vi "MasterAcquisitionFile_PCO_IOS.vi"() -> ()   [LabVIEW 2020]
uses:
  <userlib>/PCO LabVIEW 5.0.0/pco.camera/Controls/binning.ctl
  <vilib>/vision/driver/IMAQdx.llb/IMAQdx Camera Control Mode.ctl
  <vilib>/vision/driver/IMAQdx.llb/IMAQdx Acquisition Mode.ctl
  <vilib>/userDefined/High Color/IMAQdx.ctl
  <userlib>/PCO LabVIEW 5.0.0/pco.camera/Camera.lvclass
  <vilib>/vision/driver/IMAQdx.llb/IMAQdx Buffer Number Mode.ctl
  <vilib>/DAQmx/write.llb/DAQmx Write (Digital 1D Wfm NChan NSamp).vi
  <vilib>/DAQmx/write.llb/DAQmx Write (Digital Bool 1Line 1Point).vi
  <vilib>/DAQmx/read.llb/DAQmx Read (Analog 1D Wfm NChan NSamp).vi
  <vilib>/Waveform/DWDTOps.llb/DWDT Digital to Boolean Array.vi
  <vilib>/DAQmx/create/channels.llb/DAQmx Create Channel (CO-Pulse Generation-Frequency).vi
  <vilib>/DAQmx/configure/timing.llb/DAQmx Timing (Implicit).vi
  <vilib>/DAQmx/create/channels.llb/DAQmx Create Channel (AI-Voltage-Basic).vi
  <vilib>/DAQmx/configure/timing.llb/DAQmx Timing (Sample Clock).vi
  <vilib>/DAQmx/configure/trigger.llb/DAQmx Start Trigger (Digital Edge).vi
  <vilib>/DAQmx/create/channels.llb/DAQmx Create Channel (DO-Digital Output).vi
  <vilib>/Waveform/DWDTOps.llb/DWDT Boolean Array to Digital.vi
  <vilib>/Waveform/DWDTOps.llb/DWDT Uncompress Digital.vi
  <vilib>/DAQmx/miscellaneous.llb/DAQmx Fill In Error Info.vi
  <vilib>/vision/driver/NI_Vision_Acquisition_Software.lvlib
  <resource>/objmgr/imaqdx.rc
  <resource>/objmgr/daqmx.rc
panel:
  out "Recorded Images":u32=9000
  in  "ROI":cluster{"x0":u64, "y0":u64, "x1":u64, "y1":u64}={"x0"=1, "y0"=1, "x1"=640, "y1"=540}
  in  "Binning":T1={"vert"=4, "horz"=4}
  in  "TriggerMode":T2(ring)=enum."external exposure start"
  in  "Exposure [s]":dbl=0.02 min=0.0005 max=2.0 step=0.001
  out "Image":T3(plugin-control)
  out "LED":bool
  out "Auditory":bool
  out "RPad":bool
  out "LPad":bool
  out "Finished":bool=TRUE
  in  "Generate Stimuli":bool=TRUE
  in  "Sol Stim Parameters":cluster{"Fs":dbl, "Samples":dbl}
  in  "LED Stim Parameters":cluster{"Fs":dbl, "Samples":dbl}
  in  "Sol Duty Cycle (%)":dbl=50.0
  in  "Sol Freq":dbl=1.0
  in  "Sol Dur (s)":dbl=1.0
  in  "LED Duty Cycle (%)":dbl=10.0
  in  "LED Freq":dbl=10.0
  in  "LED Dur (s)":dbl=2.0
  out "Stimulus Order":digitalwaveform[](graph)=[{"t0"=timestamp(0 s since 1904-01-01), "dt"=5e-05, "Y"={"transitions"=[], "data"=array6001000x1[6001000 elements]}}, {"t0"=timestamp(0 s since 1904-01-01), "dt"=5e-05, "Y"={"transitions"=[], "data"=array6001000x1[6001000 elements]}}, {"t0"=timestamp(0 s since 1904-01-01), "dt"=5e-05, "Y"={"transitions"=[], "data"=array6001000x1[6001000 elements]}}, {"t0"=timestamp(0 s since 1904-01-01), "dt"=5e-05, "Y"={"transitions"=[], "data"=array6001000x1[6001000 elements]}}]
  out "Solenoid Stim":digitalwaveform(graph)={"t0"=timestamp(0 s since 1904-01-01), "dt"=5e-05, "Y"={"transitions"=[], "data"=array20000x1[20000 elements]}}
  in  "Trial Offset (s)":dbl=15.0
  in  "Interstim (s)":dbl=30.0
  in  "Right Pad":dbl=1.0
  in  "Left Pad":dbl=1.0
  in  "Auditory":dbl=1.0
  in  "LED":dbl
  out "?":T3(plugin-control)
  out "?":T3(plugin-control)
  out "?":T3(plugin-control)
  in  "stop":bool
  out "PCO":bool=TRUE
  out "Pupil Cam":bool=TRUE
  out "Whisk Cam":bool=TRUE
  out "Web Cam":bool=TRUE
  out "Analog":bool=TRUE
  out "Web Cam Fs":dbl(knob)=16.167664670658684 scale=0.0..200.0
  out "Whisk Cam Fs":dbl(knob)=150.0 scale=0.0..200.0
  out "Last Whisk\nBuffer 2":u32=9001
  out "Pupil Cam Fs":dbl(knob)=30.0 scale=0.0..200.0
  out "Dropped 2":u32(slide) caption="Pupil Cam" scale=0.0..99.0
  out "Dev1 Samples":i32=6000014
  in  "Dev1 Analog Channels":string[](array[string])=["Cortical_LH", "Force_Sensor", "LPadSol", "RPadSol", "AudSol", "Hippocampus", "EMG", "Cortical_RH", "OptoLED"]
  in  "Analog Acquisition":cluster{"Analog Fs":u16}={"Analog Fs"=20000} {"Analog Fs" format="%0.0f"}
  in  "Sampling Rates":T4={"CBV Cam Fs"=30, "Whisk Cam Fs"=150, "Web Cam Fs"=30, "Pupil Cam Fs"=30}
  out "Notes Size":i32=10
  out "Notes Reversed":string[](array[string])=["Experimenter", "Animal ID", "Hemisphere", "Solenoid PSI", "Isoflurane time", "Session ID", "Amplifier Gain", "Opto LED (mW)", "Wavelengths", "Lens mag"]
  out "Notes Array":string[](array[string])=["Lens mag", "Wavelengths", "Opto LED (mW)", "Amplifier Gain", "Session ID", "Isoflurane time", "Solenoid PSI", "Hemisphere", "Animal ID", "Experimenter"]
  in  "Notes:":T5={"Experimenter"="Kevin", "Animal ID"="FS28", "Hemisphere"="RH", "Solenoid PSI"="10", "Isoflurane time"="1320", "Session ID"="Imaging Session Two", "Amplifier Gain"="10000", "Opto LED (mW)"="10", "Wavelengths"="RGB", "Lens mag"="3X"}
  in  "Target Path":path=path "D:/FS28/1min_470_OptoLED_NotesTests" caption="Final Save Location"
  out "Dropped":u32(slide) caption="Whisk Cam" scale=0.0..999.0
  out "Filename":string="230407_13_50_46"
  out "CBV Camera":bool=TRUE
  out "Time Elapsed (Min)":cluster{dbl, dbl}(slide)={5.0, 5.0012167100000005} scale=0.0..15.0 scale format="%.1g"
  in  "Time (min)":dbl(knob)=5.0 min=0.5 max=20.0 step=0.5 scale=0.0..20.0 scale format="%#_2g"
  in  "Temp Path":path=path "D:/LabVIEW Streamed Data" caption="Temporary Path for Streamed Data"
  out "Last Whisk\nBuffer":u32=45001
  # "PCO Parameters"
  # "Stimuli"
  # "LPAD"
  # "RPAD"
  # "AUD"
  # "LED"
  # "Dropped Frames"
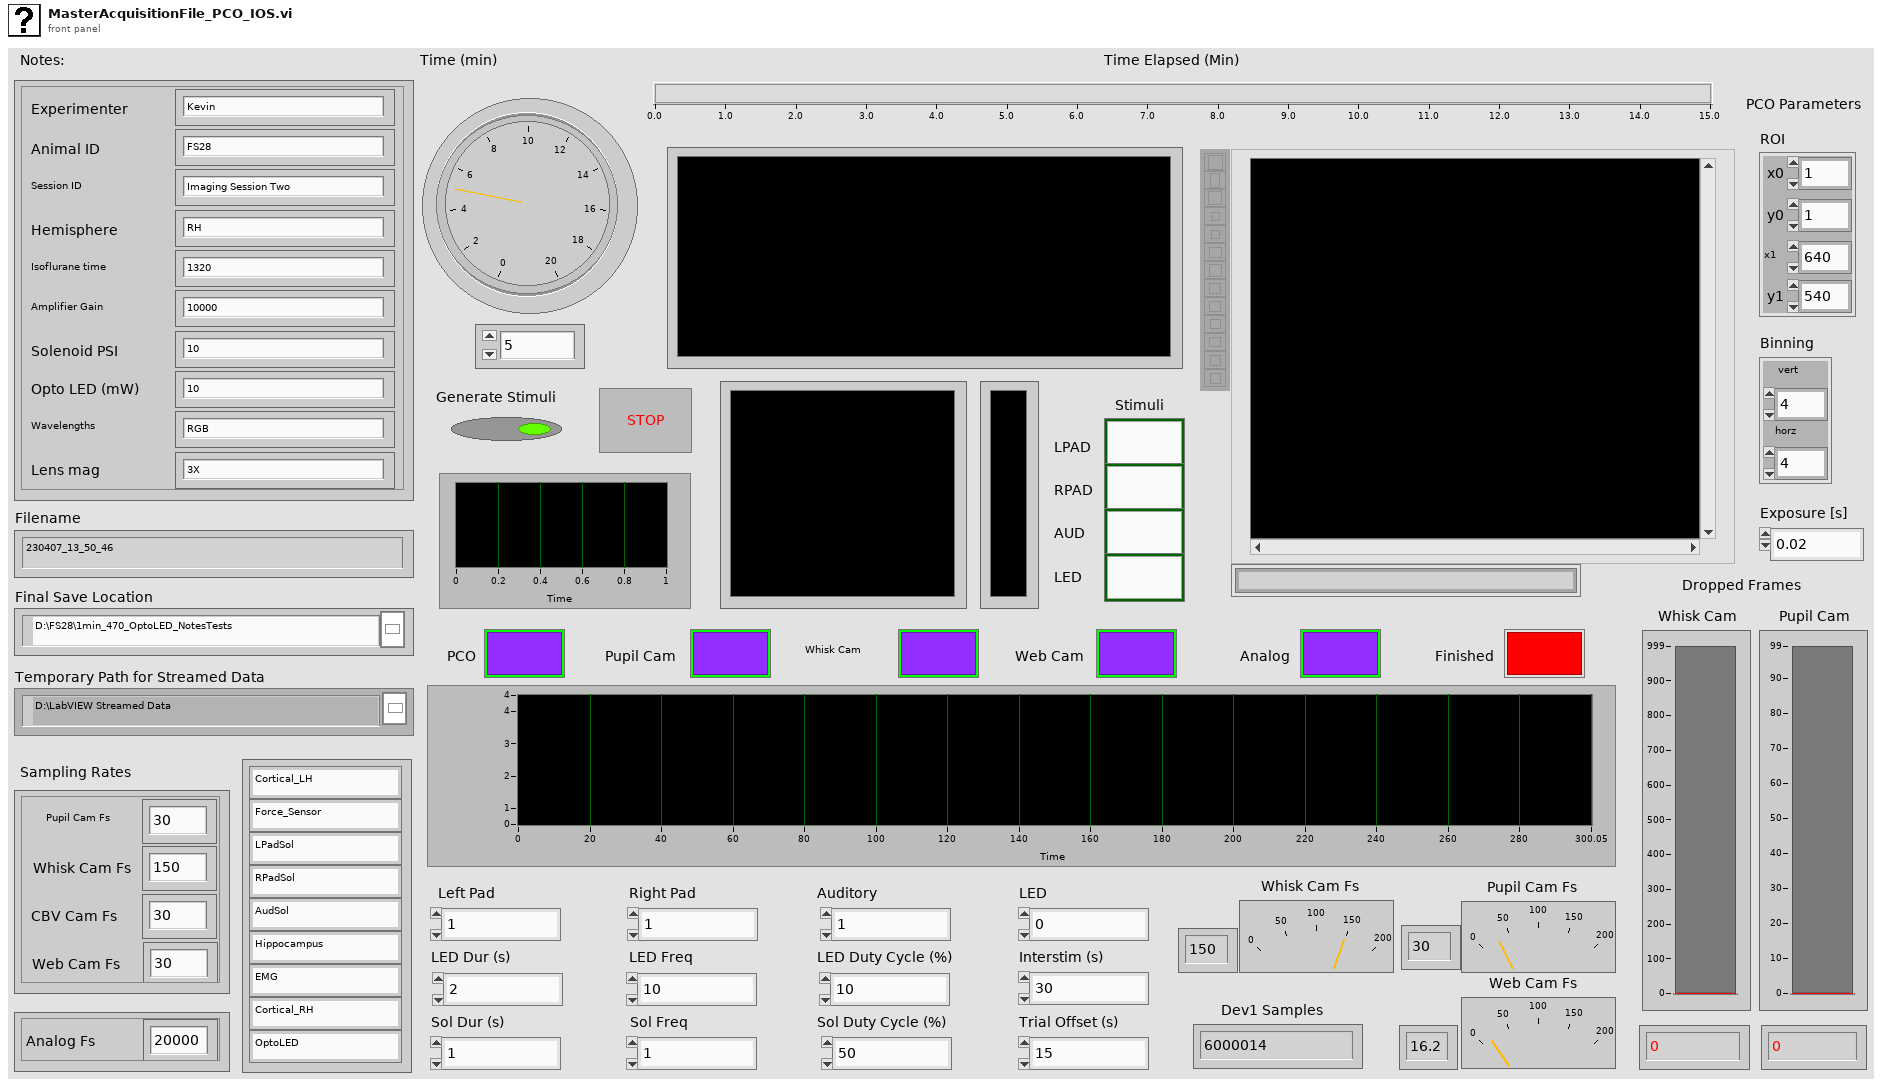
[diagram p1: front panel]
types:
  T1 = typedef "Camera.lvclass/binning.ctl" = cluster{"vert":u16, "horz":u16}
  T2 = enum16{"auto sequence", "software trigger", "external exposure start", "external exposure control"}
  T3 = typedef "IMAQ Image.ctl" = refnum<image>
  T4 = cluster{"CBV Cam Fs":u16, "Whisk Cam Fs":u16, "Web Cam Fs":u16, "Pupil Cam Fs":u16}
  T5 = cluster{"Experimenter":string, "Animal ID":string, "Hemisphere":string, "Solenoid PSI":string, "Isoflurane time":string, "Session ID":string, "Amplifier Gain":string, "Opto LED (mW)":string, "Wavelengths":string, "Lens mag":string}
  T6 = typedef "Image Type" = u32
  T7 = typedef "IMAQdx.ctl" = refnum<k21>
  T8 = enum16{"open", "replace", "create", "open or create", "replace or create", "replace or create with confirmation"}
  T9 = typedef "NI_Vision_Acquisition_Software.lvlib/IMAQdx Acquisition Mode.ctl" = enum32{"One Shot", "Continuous"}
  T10 = typedef "NI_Vision_Acquisition_Software.lvlib/IMAQdx Camera Control Mode.ctl" = enum32{"Controller", "Listener"}
  T11 = enum16{"open", "open or create", "create or replace", "create", "open (read-only)"}
  T12 = cluster{"exposure_time_s":dbl, "delay_time_s":dbl, "roi":cluster{"x0":u64, "y0":u64, "x1":u64, "y1":u64}, "timestamp_mode":u16, "pixelrate":u32, "trigger_mode":u16, "acquire_mode":u16, "metadata_mode":u16, "noisefilter_mode":u16, "binning":T1}
  T13 = typedef "IMAQ AVI2 Refnum.ctl" = refnum<k20>
  T14 = enum16{"sequence", "sequence non blocking", "ring buffer", "fifo", "sequence_dpcore", "sequence_non_blocking_dpcore", "ring_buffer_dpcore", "fifo_dpcore", "tif", "multitif", "pcoraw", "b16", "dicom", "multidicom"}
  T15 = enum16{"Undefined", "Mono8", "Mono16", "BGRA8", "RGBA8", "BGRA16", "RGBA16", "CompressedMono8"}
  T16 = enum16{"big-endian, network order", "native, host order", "little-endian"}
  T17 = typedef "NI_Vision_Acquisition_Software.lvlib/IMAQdx Buffer Number Mode.ctl" = enum32{"Next", "Last", "Buffer Number", "Every", "Last New"}
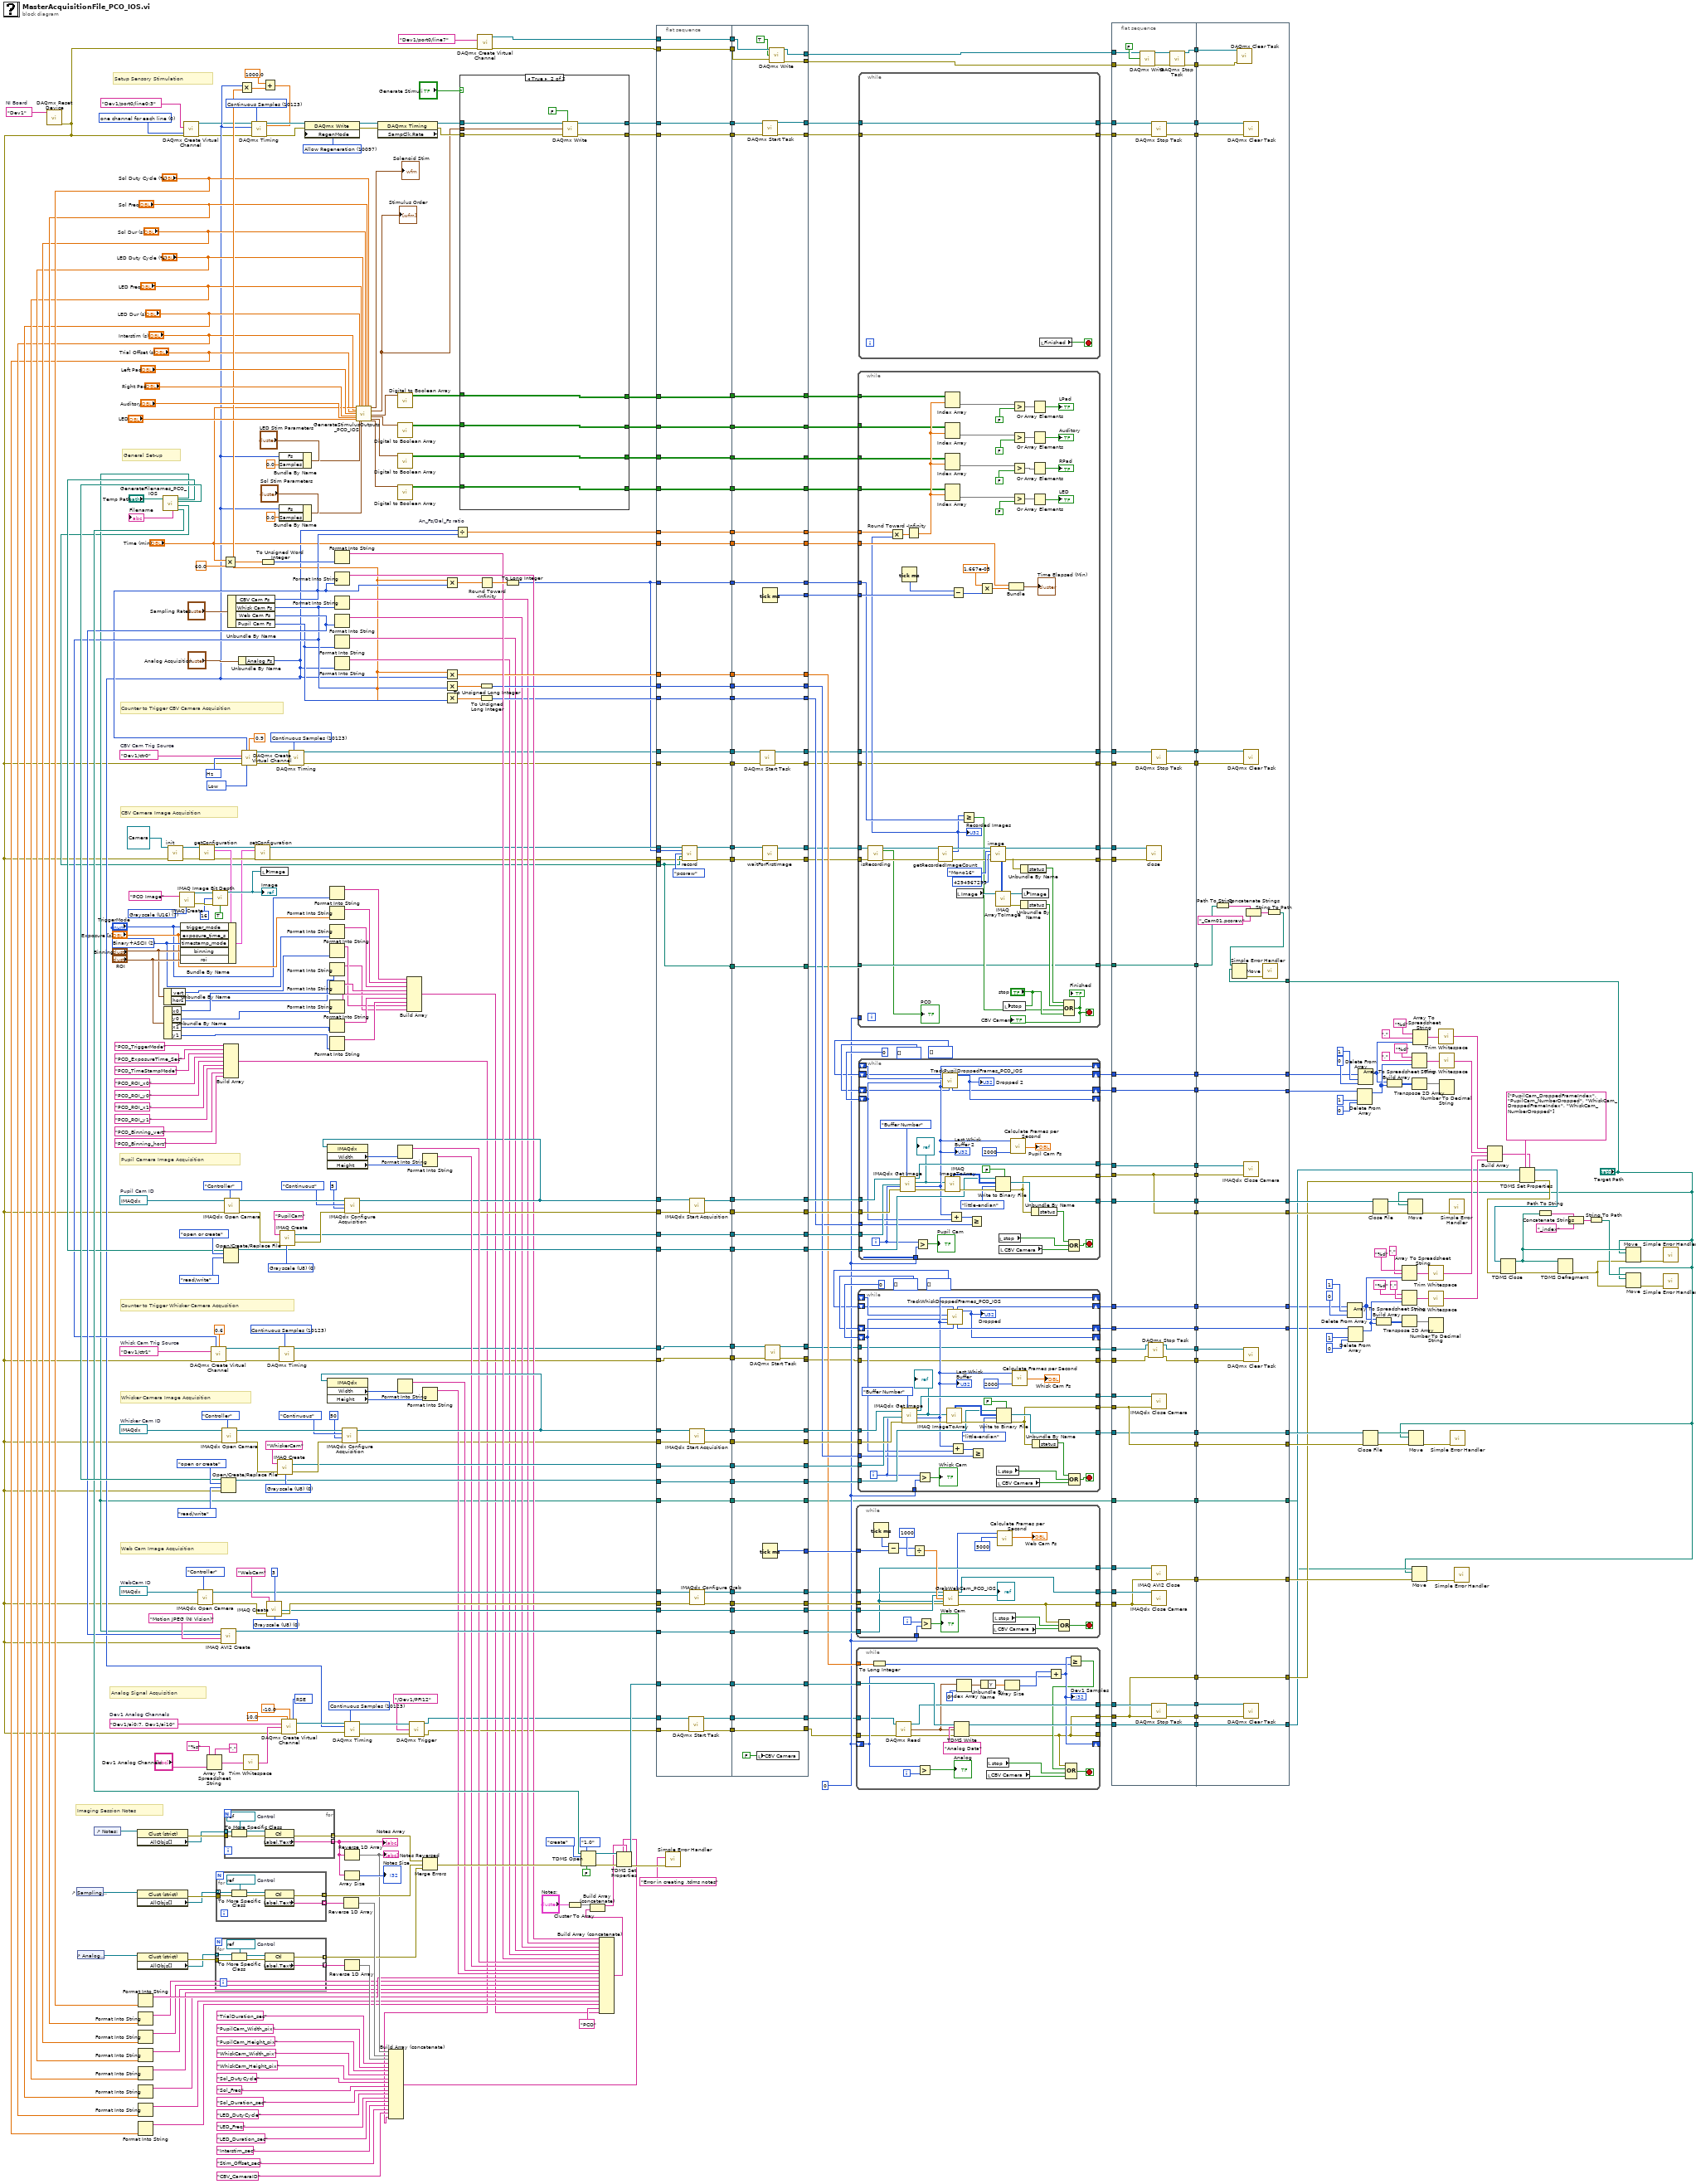
[diagram p0: block diagram]
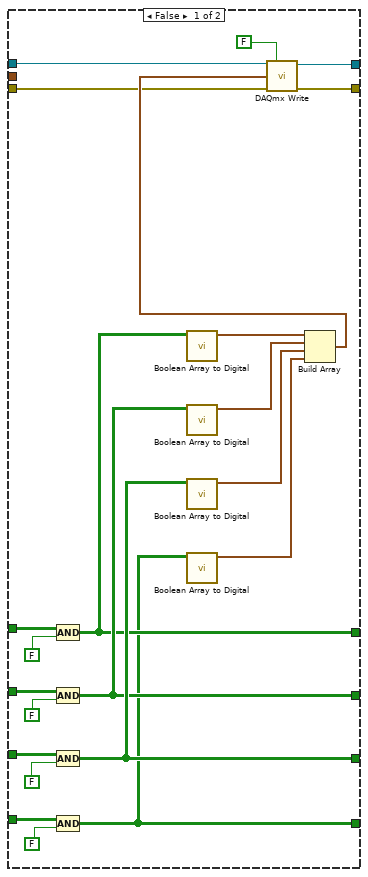
[diagram p2: hidden frame]
diagram:
  w6 = u16 2 items=["OFF", "Binary", "Binary+ASCII", "ASCII"] ("wTimeStampMode")
  w98 = T6 7 items=["Grayscale (U8)", "Grayscale (I16)", "Grayscale (SGL)", "Complex (CSG)", "RGB (U32)", "HSL (U32)", "RGB (U64)", "Grayscale (U16)"] ("Image Type")
  w179 = 10097 items=["Allow Regeneration"=10097, "Do Not Allow Regeneration"=10158] ("RegenMode")
  w180 = 10123 items=["Finite Samples"=10178, "Continuous Samples"=10123, "Hardware Timed Single Point"=12522] ("sample mode")
  w183 = 0 items=["one channel for each line", "one channel for all lines"] ("line grouping")
  w352 = tag "Dev1/ai0:7, Dev1/ai10"  # Dev1 Analog Channels
  w355 = T7 "cam3"  # WebCam ID
  w341 = T7 "cam1"  # Whisker Cam ID
  w461 = tag "Dev1/ctr1"  # Whisk Cam Trig Source
  w303 = T7 "cam2"  # Pupil Cam ID
  w152 = tag "Dev1/ctr0"  # CBV Cam Trig Source
  w306 = T6 0 items=["Grayscale (U8)", "Grayscale (I16)", "Grayscale (SGL)", "Complex (CSG)", "RGB (U32)", "HSL (U32)", "RGB (U64)", "Grayscale (U16)"] ("Image Type")
  w236 = 0
  w410 = 10123 items=["Finite Samples"=10178, "Continuous Samples"=10123, "Hardware Timed Single Point"=12522] ("sample mode")
  w413 = 10083 items=["default"=-1, "RSE"=10083, "NRSE"=10078, "Differential"=10106, "Pseudodifferential"=12529] ("input terminal configuration")
  w444 = T6 0 items=["Grayscale (U8)", "Grayscale (I16)", "Grayscale (SGL)", "Complex (CSG)", "RGB (U32)", "HSL (U32)", "RGB (U64)", "Grayscale (U16)"] ("Image Type")
  w451 = tag "Dev1"  # NI Board
  w452 = 10123 items=["Finite Samples"=10178, "Continuous Samples"=10123, "Hardware Timed Single Point"=12522] ("sample mode")
  w455 = 10373 items=["Hz"=10373] ("units")
  w456 = 10214 items=["High"=10192, "Low"=10214] ("idle state")
  w457 = 10123 items=["Finite Samples"=10178, "Continuous Samples"=10123, "Hardware Timed Single Point"=12522] ("sample mode")
  w464 = T6 0 items=["Grayscale (U8)", "Grayscale (I16)", "Grayscale (SGL)", "Complex (CSG)", "RGB (U32)", "HSL (U32)", "RGB (U64)", "Grayscale (U16)"] ("Image Type")
  # "General Set-up"
  # "Pupil Camera Image Acquisition"
  # "Whisker Camera Image Acquisition"
  # "Imaging Session Notes"
  # "Setup Sensory Stimulation"
  # "CBV Camera Image Acquisition"
  # "Counter to Trigger CBV Camera Acquisition"
  # "Counter to Trigger Whisker Camera Acqusition"
  # "Web Cam Image Acquisition"
  # "Analog Signal Acquisition"
  n1 = call <vilib>:"DAQmx Reset Device.vi"("device in"=w451) -> ("error out"=w60:errorcluster)  [unwired: 14 in]
  n2 = control-ref of="Sampling Rates"() -> (w361:refnum<vi>)
  n3 = control-ref of="Analog Acquisition"() -> (w360:refnum<vi>)
  n4 = control-ref of="Notes:"() -> (w382:refnum<vi>)
  n5 = property class="Clust (strict)"(reference=w382) -> (error out=w385:errorcluster, "AllObjs[]"=w319:refnum<vi>[])  [unwired: 1 in, 1 out]
  n6 = property class="Clust (strict)"(reference=w361) -> (error out=w380:errorcluster, "AllObjs[]"=w320:refnum<vi>[])  [unwired: 1 in, 1 out]
  n7 = property class="Clust (strict)"(reference=w360) -> (error out=w359:errorcluster, "AllObjs[]"=w318:refnum<vi>[])  [unwired: 1 in, 1 out]
  n8 = Format Into String("Sol Duty Cycle (%)") -> (resulting string=w213:string)  [unwired: 3 in, 1 out]
  n9 = Format Into String("Sol Freq") -> (resulting string=w212:string)  [unwired: 3 in, 1 out]
  n10 = Format Into String("Sol Dur (s)") -> (resulting string=w211:string)  [unwired: 3 in, 1 out]
  n11 = Format Into String("LED Duty Cycle (%)") -> (resulting string=w210:string)  [unwired: 3 in, 1 out]
  n12 = Format Into String("LED Freq") -> (resulting string=w209:string)  [unwired: 3 in, 1 out]
  n13 = Format Into String("LED Dur (s)") -> (resulting string=w208:string)  [unwired: 3 in, 1 out]
  n14 = Format Into String("Interstim (s)") -> (resulting string=w207:string)  [unwired: 3 in, 1 out]
  n15 = Format Into String("Trial Offset (s)") -> (resulting string=w206:string)  [unwired: 3 in, 1 out]
  n16 = call "GenerateFilenames_PCO_IOS.vi"("path"="Temp Path") -> ("TDMS Path"=w377:path, "PCO Path"=w68:path, "Basler Path"=w447:path, "WebCam Path"=w102:path, "Analog file name"=→"Filename":string, "Basler2 Path"=w302:path)  [unwired: 3 in, 2 out]
  n17 = Unbundle By Name("Binning") -> ("vert"=w7:u16, "horz"=w8:u16)
  n18 = Unbundle By Name("ROI") -> ("x0"=w9:u64, "y0"=w10:u64, "x1"=w11:u64, "y1"=w12:u64)
  n19 = call-dynamic "init.vi"("Camera in"=refnum<class "Camera.lvclass"> refnum ("PCOCamera in"), "error in (no error)"=w60) -> ("Camera out"=w91:refnum<class "Camera.lvclass">, "error out"=w90:errorcluster)  [unwired: 7 in]
  n20 = call "IMAQ Create"("Image Name"="PCO Image", "Image Type"=w98) -> ("New Image"=w97:T3, "error out"=w96:errorcluster)  [unwired: 3 in]
  n21 = call-poly <vilib>:"DAQmx Create Virtual Channel.vi"("lines"=tag "Dev1/port0/line0:3", "line grouping"=w183, "error in"=w60) -> ("task out"=w182:refnum<k21>, "error out"=w181:errorcluster)  [unwired: 11 in]
  n22 = call <vilib>:"IMAQdx Open Camera.vi"("Camera Control Mode"=IMAQdx_Camera_Control_Mode."Controller", "error in"=w60, "Session In"=w355) -> ("error out"=w440:errorcluster, "Session Out"=w438:T7)  [unwired: 7 in]
  n23 = call-dynamic "getConfiguration.vi"("error in (no error)"=w90, "Camera in"=w91) -> ("error out"=w89:errorcluster, "configuration"=w93:T12, "Camera out"=w92:refnum<class "Camera.lvclass">)  [unwired: 7 in]
  n24 = Bundle By Name(cluster=w93, "trigger_mode"="TriggerMode", "exposure_time_s"="Exposure [s]", "timestamp_mode"=w6, "binning"="Binning", "roi"="ROI") -> (w88:T12)
  n25 = Array To Spreadsheet String(delimiter (Tab)=",", array="Dev1 Analog Channels", 3:"%s" ("format string")) -> (spreadsheet string=w349:string)
  n26 = call "IMAQ Image Bit Depth"("Image"=w97, "Bit Depth (0)"=u32 16, "error in (no error)"=w96, "Get/Set Bit Depth? (Set)"=TRUE) -> ("Image Out"=w99:T3)  [unwired: 9 in, 2 out]
  "Image" <- w99
  n27 = for {
    tunnel: [w476] -> w357 mode=indexing
    tunnel: w359 -> [w475]
    tunnel: [w473] -> w358 mode=indexing
    tunnel: w318 -> [w472] mode=indexing
    w477 = refnum<vi> refnum  # Control
    n28 = To More Specific Class(target class=w477, reference=w472, error in=w475) -> (specific class reference=w478:refnum<vi>, error out=w474:errorcluster)
    n29 = property class="Ctl"(reference=w478, error in=w474) -> (error out=w473:errorcluster, "Label.Text"=w476:string)  [unwired: 1 out]
  }
  n30 = for {
    tunnel: [w483] -> w381 mode=indexing
    tunnel: w380 -> [w482]
    tunnel: [w480] -> w367 mode=indexing
    tunnel: w320 -> [w479] mode=indexing
    w484 = refnum<vi> refnum  # Control
    n31 = To More Specific Class(target class=w484, reference=w479, error in=w482) -> (specific class reference=w485:refnum<vi>, error out=w481:errorcluster)
    n32 = property class="Ctl"(reference=w485, error in=w481) -> (error out=w480:errorcluster, "Label.Text"=w483:string)  [unwired: 1 out]
  }
  n33 = Open/Create/Replace File(file path (use dialog)=w447, error in=w60, operation (0:open)=T8."open or create", access (0:read/write)=enum16{"read/write", "read-only", "write-only"}."read/write") -> (refnum out=w419:refnum<file>)  [unwired: 2 in, 2 out]
  n34 = call <vilib>:"IMAQdx Open Camera.vi"("Camera Control Mode"=IMAQdx_Camera_Control_Mode."Controller", "error in"=w60, "Session In"=w341) -> ("error out"=w467:errorcluster, "Session Out"=w470:T7)  [unwired: 7 in]
  n35 = Multiply(x="Time (min)", y=60.0) -> (x*y=w223:dbl)
  n36 = Build Array("PCO_TriggerMode", "PCO_ExposureTime_Sec", "PCO_TimeStampMode", "PCO_ROI_x0", "PCO_ROI_y0", "PCO_ROI_x1", "PCO_ROI_y1", "PCO_Binning_vert", "PCO_Binning_horz") -> (w20:string[])
  n37 = Open/Create/Replace File(file path (use dialog)=w302, operation (0:open)=T8."open or create", access (0:read/write)=enum16{"read/write", "read-only", "write-only"}."read/write") -> (refnum out=w287:refnum<file>)  [unwired: 3 in, 2 out]
  n38 = call <vilib>:"IMAQdx Open Camera.vi"("Camera Control Mode"=IMAQdx_Camera_Control_Mode."Controller", "error in"=w60, "Session In"=w303) -> ("error out"=w309:errorcluster, "Session Out"=w312:T7)  [unwired: 7 in]
  n39 = for {
    tunnel: [w490] -> w384 mode=indexing
    tunnel: w385 -> [w489]
    tunnel: [w487] -> w368 mode=indexing
    tunnel: w319 -> [w486] mode=indexing
    w491 = refnum<vi> refnum  # Control
    n40 = To More Specific Class(target class=w491, reference=w486, error in=w489) -> (specific class reference=w492:refnum<vi>, error out=w488:errorcluster)
    n41 = property class="Ctl"(reference=w492, error in=w488) -> (error out=w487:errorcluster, "Label.Text"=w490:string)  [unwired: 1 out]
  }
  "Notes Array" <- w384
  n42 = Unbundle By Name("Sampling Rates") -> ("CBV Cam Fs"=w224:u16, "Whisk Cam Fs"=w276:u16, "Web Cam Fs"=w354:u16, "Pupil Cam Fs"=w270:u16)
  n43 = call-poly <vilib>:"DAQmx Create Virtual Channel.vi"("frequency"=w276, "duty cycle"=0.6, "counter"=w461, "error in"=w60) -> ("task out"=w459:refnum<k21>, "error out"=w458:errorcluster)  [unwired: 10 in]
  n44 = call "IMAQ AVI2 Create"("error in (no error)"=w60, "Codec"="Motion JPEG (NI Vision)", "Frames Per Second"=w354, "AVI Path"=w102) -> ("AVI Refnum"=w430:T13)  [unwired: 6 in, 1 out]
  n45 = Unbundle By Name("Analog Acquisition") -> ("Analog Fs"=w196:u16)
  n46 = Multiply(x=w196, y=w223) -> (x*y=w161:dbl)
  n47 = call-poly <vilib>:"DAQmx Create Virtual Channel.vi"("frequency"=w224, "duty cycle"=0.9, "counter"=w152, "units"=w455, "error in"=w60, "idle state"=w456) -> ("task out"=w454:refnum<k21>, "error out"=w453:errorcluster)  [unwired: 8 in]
  n48 = call <vilib>:"Trim Whitespace.vi"("string"=w349) -> ("trimmed string"=w348:string)  [unwired: 1 in]
  n49 = call-dynamic "setConfiguration.vi"("error in (no error)"=w89, "configuration"=w88, "Camera in"=w92) -> ("error out"=w72:errorcluster, "Camera out"=w71:refnum<class "Camera.lvclass">)  [unwired: 7 in]
  n50 = To Unsigned Word Integer(number=w223) -> (unsigned 16bit integer=w344:u16)
  n51 = local write "Image"(w99) -> ()
  n52 = Add(x=1000.0, y=w161) -> (x+y=w159:dbl)
  n53 = call-poly <vilib>:"DAQmx Timing.vi"("task/channels in"=w182, "sample mode"=w180, "samples per channel"=w159, "rate"=w196, "error in"=w181) -> ("task out"=w176:refnum<k21>, "error out"=w175:errorcluster)  [unwired: 9 in]
  n54 = call "IMAQ Create"("Border Size"=3, "Image Name"="WebCam", "Image Type"=w444, "error in (no error)"=w440) -> ("New Image"=w437:T3, "error out"=w439:errorcluster)  [unwired: 1 in]
  n55 = call "IMAQ Create"("Image Name"="WhiskerCam", "Image Type"=w464, "error in (no error)"=w467) -> ("New Image"=w339:T3, "error out"=w465:errorcluster)  [unwired: 2 in]
  n56 = Bundle By Name(cluster="LED Stim Parameters", "Fs"=w196, "Samples"=0.0) -> (w229:cluster{"Fs":dbl, "Samples":dbl})
  n57 = Bundle By Name(cluster="Sol Stim Parameters", "Fs"=w196, "Samples"=0.0) -> (w230:cluster{"Fs":dbl, "Samples":dbl})
  n58 = call-poly <vilib>:"DAQmx Timing.vi"("task/channels in"=w459, "sample mode"=w457, "error in"=w458) -> ("task out"=w35:refnum<k21>, "error out"=w37:errorcluster)  [unwired: 11 in]
  n59 = call "IMAQ Create"("Image Name"="PupilCam", "Image Type"=w306, "error in (no error)"=w309) -> ("New Image"=w279:T3, "error out"=w307:errorcluster)  [unwired: 2 in]
  n60 = call-poly <vilib>:"DAQmx Create Virtual Channel.vi"("maximum value"=10.0, "minimum value"=-10.0, "input terminal configuration"=w413, "physical channels"=w352, "name to assign"=w348, "error in"=w60) -> ("task out"=w412:refnum<k21>, "error out"=w411:errorcluster)  [unwired: 8 in]
  n61 = call-poly <vilib>:"DAQmx Timing.vi"("task/channels in"=w454, "sample mode"=w452, "error in"=w453) -> ("task out"=w44:refnum<k21>, "error out"=w42:errorcluster)  [unwired: 11 in]
  n62 = property class="DAQmx Write"(reference=w176, error in=w175, "RegenMode"=w179) -> (reference out=w177:refnum<k21>, error out=w178:errorcluster)
  n63 = Format Into String("TriggerMode") -> (resulting string=w19:string)  [unwired: 3 in, 1 out]
  n64 = Format Into String("Exposure [s]") -> (resulting string=w18:string)  [unwired: 3 in, 1 out]
  n65 = Format Into String(w6) -> (resulting string=w17:string)  [unwired: 3 in, 1 out]
  n66 = Format Into String(w7) -> (resulting string=w2:string)  [unwired: 3 in, 1 out]
  n67 = Format Into String(w8) -> (resulting string=w1:string)  [unwired: 3 in, 1 out]
  n68 = Format Into String(w9) -> (resulting string=w16:string)  [unwired: 3 in, 1 out]
  n69 = Format Into String(w10) -> (resulting string=w15:string)  [unwired: 3 in, 1 out]
  n70 = Format Into String(w11) -> (resulting string=w14:string)  [unwired: 3 in, 1 out]
  n71 = Format Into String(w12) -> (resulting string=w13:string)  [unwired: 3 in, 1 out]
  n72 = Format Into String(w344) -> (resulting string=w346:string)  [unwired: 3 in, 1 out]
  n73 = Format Into String(w224) -> (resulting string=w274:string)  [unwired: 3 in, 1 out]
  n74 = Format Into String(w276) -> (resulting string=w273:string)  [unwired: 3 in, 1 out]
  n75 = Format Into String(w354) -> (resulting string=w272:string)  [unwired: 3 in, 1 out]
  n76 = Format Into String(w270) -> (resulting string=w241:string)  [unwired: 3 in, 1 out]
  n77 = Format Into String(w196) -> (resulting string=w240:string)  [unwired: 3 in, 1 out]
  n78 = call <vilib>:"IMAQdx Configure Acquisition.vi"("error in"=w465, "Number of Buffers"=u32 50, "Continuous?"=IMAQdx_Acquisition_Mode."Continuous", "Session In"=w470) -> ("error out"=w248:errorcluster, "Session Out"=w340:T7)  [unwired: 6 in]
  n79 = property class="IMAQdx"(reference=w340) -> ("Width"=w343:u32, "Height"=w342:u32)  [unwired: 1 in, 2 out]
  n80 = Reverse 1D Array(array=w381) -> (reversed array=w371:string[])
  n81 = Reverse 1D Array(array=w384) -> (reversed array=w317:string[])
  "Notes Reversed" <- w317
  n82 = Array Size(array=w384) -> (size(s)=→"Notes Size":i32)
  n83 = Reverse 1D Array(array=w357) -> (reversed array=w356:string[])
  n84 = call <vilib>:"IMAQdx Configure Acquisition.vi"("error in"=w307, "Number of Buffers"=u32 5, "Continuous?"=IMAQdx_Acquisition_Mode."Continuous", "Session In"=w312) -> ("error out"=w289:errorcluster, "Session Out"=w280:T7)  [unwired: 6 in]
  n85 = property class="IMAQdx"(reference=w280) -> ("Width"=w301:u32, "Height"=w300:u32)  [unwired: 1 in, 2 out]
  n86 = call-poly <vilib>:"DAQmx Timing.vi"("task/channels in"=w412, "sample mode"=w410, "rate"=w196, "error in"=w411) -> ("task out"=w316:refnum<k21>, "error out"=w409:errorcluster)  [unwired: 10 in]
  n87 = call "GenerateStimulusOutputs_PCO_IOS.vi"("Trial duration (min)"="Time (min)", "Rest duration(s)"="Interstim (s)", "trial offset (s)"="Trial Offset (s)", "Left Pad"="Left Pad", "Right Pad"="Right Pad", "Auditory"="Auditory", "LED"="LED", "LED Stim Duration (s)"="LED Dur (s)", "LED Stim Parameters"=w229, "LED Frequency"="LED Freq", "Sol Stim Parameters"=w230, "LED duty cycle (%)"="LED Duty Cycle (%)", "Sol Stim Duration (s)"="Sol Dur (s)", "Sol Frequency"="Sol Freq", "Sol Duty Cycle (%)"="Sol Duty Cycle (%)") -> ("Solenoid Stim Waveforms"=→"Solenoid Stim":digitalwaveform, "Stimulus Digital Outputs"=w162:digitalwaveform[], "Left Pad Out"=w187:digitalwaveform, "Auditory Out"=w186:digitalwaveform, "Right Pad Out"=w185:digitalwaveform, "LED Out"=w184:digitalwaveform)  [unwired: 7 in]
  "Stimulus Order" <- w162
  n88 = property class="DAQmx Timing" props=["SampClk.Rate"](reference=w177, error in=w178) -> (reference out=w27:refnum<k21>, error out=w173:errorcluster)  [unwired: 1 out]
  n89 = Build Array (concatenate)(w317, w371, w356, "TrialDuration_sec", "PupilCam_Width_pix", "PupilCam_Height_pix", "WhiskCam_Width_pix", "WhiskCam_Height_pix", "Sol_DutyCycle", "Sol_Freq", "Sol_Duration_sec", "LED_DutyCycle", "LED_Freq", "LED_Duration_sec", "Interstim_sec", "Stim_Offset_sec", "CBV_CameraID", w20) -> (w314:string[])
  n90 = Format Into String(w301) -> (resulting string=w292:string)  [unwired: 3 in, 1 out]
  n91 = Format Into String(w343) -> (resulting string=w294:string)  [unwired: 3 in, 1 out]
  n92 = call-poly <vilib>:"Digital to Boolean Array.vi"("digital waveform"=w187) -> ("boolean array"=w170:bool[][])  [unwired: 9 in, 1 out]
  n93 = call-poly <vilib>:"Digital to Boolean Array.vi"("digital waveform"=w186) -> ("boolean array"=w169:bool[][])  [unwired: 9 in, 1 out]
  n94 = call-poly <vilib>:"Digital to Boolean Array.vi"("digital waveform"=w185) -> ("boolean array"=w168:bool[][])  [unwired: 9 in, 1 out]
  n95 = call-poly <vilib>:"Digital to Boolean Array.vi"("digital waveform"=w184) -> ("boolean array"=w167:bool[][])  [unwired: 9 in, 1 out]
  n96 = Build Array(w19, w18, w17, w16, w15, w14, w13, w2, w1) -> (w3:string[])
  n97 = call-poly <vilib>:"DAQmx Trigger.vi"("task/channels in"=w316, "source"=tag "/Dev1/PFI12", "error in"=w409) -> ("task out"=w33:refnum<k21>, "error out"=w32:errorcluster)  [unwired: 11 in]
  n98 = Format Into String(w300) -> (resulting string=w293:string)  [unwired: 3 in, 1 out]
  n99 = Format Into String(w342) -> (resulting string=w295:string)  [unwired: 3 in, 1 out]
  n100 = Merge Errors(w368, w367, w358) -> (w366:errorcluster)
  n101 = Multiply(x=w223, y=w224) -> (x*y=w449:dbl)
  n102 = Multiply(x=w223, y=w196) -> (x*y=w330:dbl)
  n103 = Multiply(x=w276, y=w223) -> (x*y=w315:dbl)
  n104 = Multiply(x=w270, y=w223) -> (x*y=w275:dbl)
  n105 = Divide "An_Fs/Dal_Fs ratio"(x=w196, y=w224) -> (x/y=w147:dbl)
  n106 = case shown="True" "Generate Stimuli" {
    tunnel: w173 -> [w503 w524]
    tunnel: [w501 w523] -> w25
    tunnel: [w502 w522] -> w23
    tunnel: w170 -> [w511 w521]
    tunnel: w169 -> [w512 w520]
    tunnel: w168 -> [w513 w519]
    tunnel: w167 -> [w514 w518]
    tunnel: [w496 w521] -> w166
    tunnel: [w497 w520] -> w165
    tunnel: [w498 w519] -> w164
    tunnel: [w494 w518] -> w163
    tunnel: w162 -> [_ w517]
    tunnel: w27 -> [w493 w515]
    frame False {
      n107 = Compound Arithmetic op=AND(w511, FALSE) -> (w496:bool[][])
      n108 = Compound Arithmetic op=AND(w512, FALSE) -> (w497:bool[][])
      n109 = Compound Arithmetic op=AND(w513, FALSE) -> (w498:bool[][])
      n110 = Compound Arithmetic op=AND(w514, FALSE) -> (w494:bool[][])
      n111 = call-poly <vilib>:"Boolean Array to Digital.vi"("boolean array"=w496) -> ("digital waveform"=w505:digitalwaveform)  [unwired: 9 in, 1 out]
      n112 = call-poly <vilib>:"Boolean Array to Digital.vi"("boolean array"=w497) -> ("digital waveform"=w500:digitalwaveform)  [unwired: 9 in, 1 out]
      n113 = call-poly <vilib>:"Boolean Array to Digital.vi"("boolean array"=w498) -> ("digital waveform"=w499:digitalwaveform)  [unwired: 9 in, 1 out]
      n114 = call-poly <vilib>:"Boolean Array to Digital.vi"("boolean array"=w494) -> ("digital waveform"=w495:digitalwaveform)  [unwired: 9 in, 1 out]
      n115 = Build Array(w505, w500, w499, w495) -> (w504:digitalwaveform[])
      n116 = call-poly <vilib>:"DAQmx Write.vi"("task/channels in"=w493, "auto start"=FALSE, "data"=w504, "error in"=w503) -> ("task out"=w501:refnum<k21>, "error out"=w502:errorcluster)  [unwired: 9 in, 1 out]
    }
    frame True {
      n117 = call-poly <vilib>:"DAQmx Write.vi"("task/channels in"=w515, "auto start"=FALSE, "data"=w517, "error in"=w524) -> ("task out"=w523:refnum<k21>, "error out"=w522:errorcluster)  [unwired: 9 in, 1 out]
    }
  }
  n118 = call-poly <vilib>:"DAQmx Create Virtual Channel.vi"("lines"=tag "Dev1/port0/line7", "error in"=w60) -> ("task out"=w56:refnum<k21>, "error out"=w59:errorcluster)  [unwired: 12 in]
  n119 = To Unsigned Long Integer(number=w315) -> (unsigned 32bit integer=w328:u32)
  n120 = To Unsigned Long Integer(number=w275) -> (unsigned 32bit integer=w271:u32)
  n121 = Round Toward -Infinity(1:w449) -> (0:w448:dbl)
  n122 = To Long Integer(number=w448) -> (32bit integer=w70:i32)
  n123 = Cluster To Array(cluster="Notes:") -> (array=w378:string[])
  n124 = TDMS Open(6:FALSE ("disable buffering? (T)"), 7:enum16{"1.0", "2.0"}."1.0" ("file format version (2.0)"), 8:w366, 10:T11."create" ("operation (0:open)"), 11:w377) -> (0:w372:errorcluster, 3:w373:refnum<k34>)  [unwired: 2 in]
  n125 = Build Array (concatenate)(w274, w273, w272, w241, w240, w346, w292, w293, w294, w295, w213, w212, w211, w210, w209, w208, w207, w206, "PCO" ("element"), w3) -> (w353:string[])
  n126 = Build Array (concatenate)(w378, w353) -> (w370:string[])
  n127 = TDMS Set Properties(5:w370, 7:w314, 8:w372, 11:w373) -> (0:w365:errorcluster, 3:w369:refnum<k34>)  [unwired: 2 in, 2 out]
  n128 = flat-sequence {
    tunnel: w439 -> [w573]
    tunnel: w438 -> [w572]
    tunnel: w437 -> [w571]
    tunnel: [w571] -> w436
    tunnel: [w570] -> w434
    tunnel: [w569] -> w432
    tunnel: w430 -> [w568]
    tunnel: [w568] -> w429
    tunnel: w340 -> [w567]
    tunnel: w248 -> [w566]
    tunnel: [w565] -> w426
    tunnel: [w564] -> w424
    tunnel: [w563] -> w422
    tunnel: w339 -> [w563]
    tunnel: [w562] -> w420
    tunnel: w419 -> [w562]
    tunnel: w70 -> [w561]
    tunnel: [w561] -> w417
    tunnel: "Time (min)" -> [w560]
    tunnel: [w560] -> w414
    tunnel: [w559] -> w407
    tunnel: w369 -> [w559]
    tunnel: w330 -> [w558]
    tunnel: [w558] -> w329
    tunnel: w328 -> [w557]
    tunnel: [w557] -> w327
    tunnel: [w552] -> w291
    tunnel: w280 -> [w553]
    tunnel: [w550] -> w290
    tunnel: w289 -> [w551]
    tunnel: [w556] -> w288
    tunnel: w287 -> [w556]
    tunnel: w279 -> [w555]
    tunnel: [w555] -> w278
    tunnel: w271 -> [w554]
    tunnel: [w554] -> w269
    tunnel: [w549] -> w195
    tunnel: w166 -> [w549]
    tunnel: [w548] -> w194
    tunnel: w165 -> [w548]
    tunnel: [w547] -> w193
    tunnel: w164 -> [w547]
    tunnel: [w546] -> w192
    tunnel: w163 -> [w546]
    tunnel: w147 -> [w545]
    tunnel: [w545] -> w146
    tunnel: w102 -> [w544]
    tunnel: [w544] -> w103
    tunnel: [w543] -> w76
    tunnel: [w542] -> w75
    tunnel: w72 -> [w540]
    tunnel: w71 -> [w539]
    tunnel: w70 -> [w538]
    tunnel: w68 -> [w537]
    tunnel: [w537] -> w65
    tunnel: w59 -> [w536]
    tunnel: [w536] -> w58
    tunnel: [w535] -> w57
    tunnel: w56 -> [w535]
    tunnel: w44 -> [w534]
    tunnel: [w534] -> w45
    tunnel: w42 -> [w533]
    tunnel: [w533] -> w43
    tunnel: w37 -> [w532]
    tunnel: [w532] -> w36
    tunnel: w35 -> [w531]
    tunnel: [w531] -> w34
    tunnel: w33 -> [w530]
    tunnel: w32 -> [w529]
    tunnel: [w528] -> w31
    tunnel: [w527] -> w30
    tunnel: [w526] -> w26
    tunnel: w25 -> [w526]
    tunnel: [w525] -> w24
    tunnel: w23 -> [w525]
    tunnel: [w624] -> w441
    tunnel: w436 -> [w623]
    tunnel: [w623] -> w435
    tunnel: w434 -> [w622]
    tunnel: [w622] -> w433
    tunnel: w432 -> [w621]
    tunnel: [w621] -> w431
    tunnel: w429 -> [w620]
    tunnel: [w620] -> w428
    tunnel: [w619] -> w427
    tunnel: w426 -> [w619]
    tunnel: [w618] -> w425
    tunnel: w424 -> [w618]
    tunnel: [w617] -> w423
    tunnel: w422 -> [w617]
    tunnel: [w616] -> w421
    tunnel: w420 -> [w616]
    tunnel: [w615] -> w418
    tunnel: w417 -> [w614]
    tunnel: [w614] -> w416
    tunnel: [w613] -> w415
    tunnel: w414 -> [w613]
    tunnel: [w612] -> w238
    tunnel: w407 -> [w612]
    tunnel: w329 -> [w611]
    tunnel: [w611] -> w239
    tunnel: w327 -> [w610]
    tunnel: [w610] -> w268
    tunnel: w291 -> [w608]
    tunnel: w290 -> [w607]
    tunnel: w288 -> [w606]
    tunnel: [w608] -> w283
    tunnel: [w607] -> w282
    tunnel: [w606] -> w281
    tunnel: [w605] -> w277
    tunnel: w278 -> [w605]
    tunnel: [w604] -> w267
    tunnel: w269 -> [w604]
    tunnel: w195 -> [w600]
    tunnel: w194 -> [w603]
    tunnel: w193 -> [w602]
    tunnel: w192 -> [w601]
    tunnel: [w600] -> w191
    tunnel: [w603] -> w190
    tunnel: [w602] -> w189
    tunnel: [w601] -> w188
    tunnel: [w585] -> w172
    tunnel: [w584] -> w171
    tunnel: w146 -> [w599]
    tunnel: [w599] -> w145
    tunnel: [w598] -> w105
    tunnel: w103 -> [w598]
    tunnel: w76 -> [w597]
    tunnel: w75 -> [w596]
    tunnel: [w595] -> w74
    tunnel: [w594] -> w73
    tunnel: [w593] -> w64
    tunnel: w65 -> [w593]
    tunnel: w58 -> [w590]
    tunnel: w57 -> [w592]
    tunnel: [w589] -> w53
    tunnel: [w588] -> w52
    tunnel: [w586] -> w49
    tunnel: [w587] -> w51
    tunnel: [w578] -> _
    tunnel: [w579] -> _
    tunnel: w45 -> [w583]
    tunnel: w43 -> [w582]
    tunnel: [w581] -> w41
    tunnel: [w580] -> w40
    tunnel: w36 -> [w579]
    tunnel: w34 -> [w578]
    tunnel: [w577] -> w28
    tunnel: w31 -> [w577]
    tunnel: [w576] -> w29
    tunnel: w30 -> [w576]
    tunnel: w26 -> [w575]
    tunnel: w24 -> [w574]
    frame #0 {
      n129 = call-dynamic "record.vi"("Camera in"=w539, "num_images"=w538, "record_mode"=T14."pcoraw", "file_path"=w537, "error in (no error)"=w540) -> ("Camera out"=w543:refnum<class "Camera.lvclass">, "error out"=w542:errorcluster)  [unwired: 9 in]
      n130 = call <vilib>:"DAQmx Start Task.vi"("task/channels in"=w530, "error in"=w529) -> ("task out"=w528:refnum<k21>, "error out"=w527:errorcluster)  [unwired: 12 in]
      n131 = call <vilib>:"IMAQdx Start Acquisition.vi"("error in"=w551, "Session In"=w553) -> ("error out"=w550:errorcluster, "Session Out"=w552:T7)  [unwired: 8 in]
      n132 = call <vilib>:"IMAQdx Start Acquisition.vi"("error in"=w566, "Session In"=w567) -> ("error out"=w564:errorcluster, "Session Out"=w565:T7)  [unwired: 8 in]
      n133 = call <vilib>:"IMAQdx Configure Grab.vi"("error in"=w573, "Session In"=w572) -> ("error out"=w569:errorcluster, "Session Out"=w570:T7)  [unwired: 8 in]
    }
    frame #1 {
      n134 = local write "CBV Camera"(FALSE ("Finished Acquiring")) -> ()
      n135 = call <vilib>:"DAQmx Start Task.vi"("task/channels in"=w583, "error in"=w582) -> ("task out"=w580:refnum<k21>, "error out"=w581:errorcluster)  [unwired: 12 in]
      n136 = call-dynamic "waitForFirstImage.vi"("error in (no error)"=w596, "Camera in"=w597) -> ("error out"=w594:errorcluster, "Camera out"=w595:refnum<class "Camera.lvclass">)  [unwired: 8 in]
      n137 = call <vilib>:"DAQmx Start Task.vi"("task/channels in"=w575, "error in"=w574) -> ("task out"=w585:refnum<k21>, "error out"=w584:errorcluster)  [unwired: 12 in]
      n138 = Tick Count (ms)() -> (millisecond timer value=w615:u32)
      n139 = Tick Count (ms)() -> (millisecond timer value=w624:u32)
      n140 = call <vilib>:"DAQmx Start Task.vi"("task/channels in"=w578, "error in"=w579) -> ("task out"=w587:refnum<k21>, "error out"=w586:errorcluster)  [unwired: 12 in]
      n141 = call-poly <vilib>:"DAQmx Write.vi"("task/channels in"=w592, "data"=TRUE, "error in"=w590) -> ("task out"=w589:refnum<k21>, "error out"=w588:errorcluster)  [unwired: 10 in, 1 out]
    }
  }
  n142 = call <vilib>:"Simple Error Handler.vi"("error source (\" \")"="Error in creating .tdms notes" ("error source (\" \")"), "error in (no error)"=w365) -> ()  [unwired: 3 in, 5 out]
  n143 = while {
    tunnel: w238 -> [w647]
    tunnel: [w646] -> w120
    tunnel: [w635] -> _
    tunnel: [w645] -> w144
    shift-right: [w639] -> _
    shift-left: w236 -> [w630]
    tunnel: [w635] -> w143
    tunnel: w239 -> [w633]
    tunnel: w29 -> [w626]
    tunnel: w28 -> [w625]
    i -> [w631]
    stop <- w636 stop-if-true
    n144 = To Long Integer(number=w633) -> (32bit integer=w634:i32)
    n145 = call-poly <vilib>:"DAQmx Read.vi"("task/channels in"=w625, "error in"=w626) -> ("task out"=w645:refnum<k21>, "data"=w627:waveform(dbl)[], "error out"=w638:errorcluster)  [unwired: 11 in]
    n146 = Greater?(x=w630, y=w631) -> (0:→"Analog":bool)
    n147 = TDMS Write(0:w647, 5:"Analog Data" ("group name in (Untitled)"), 9:w627, 11:w638) -> (4:w646:refnum<k34>, 15:w635:errorcluster)  [unwired: 2 in, 2 out]
    n148 = Index Array(array=w627, index=0) -> (element=w642:waveform(dbl))
    n149 = Unbundle By Name(w642) -> ("Y"=w641:dbl[])
    n150 = local read "CBV Camera"() -> (w629:bool)
    n151 = local read "stop"() -> (w628:bool)
    n152 = Array Size(array=w641) -> (size(s)=w640:i32)
    n153 = Add(x=w640, y=w630) -> (x+y=w639:i32)
    "Dev1 Samples" <- w639
    n154 = Greater Or Equal?(x=w639, y=w634) -> (x >= y?=w637:bool)
    n155 = Compound Arithmetic op=OR(w635, w637, w628, w629) -> (w636:bool)
  }
  n156 = while {
    tunnel: w441 -> [w664]
    tunnel: w435 -> [w662]
    tunnel: w433 -> [w661]
    tunnel: w431 -> [w660]
    tunnel: w428 -> [w658]
    tunnel: [w659] -> w139
    tunnel: [w650] -> w140
    tunnel: [w658] -> w138
    tunnel: w236 -> [w653]
    i -> [w654]
    stop <- w651 stop-if-true
    n157 = Tick Count (ms)() -> (millisecond timer value=w666:u32)
    n158 = Subtract(x=w666, y=w664) -> (x-y=w667:u32)
    n159 = Divide(x=w667, y=u32 1000) -> (x/y=w663:dbl)
    n160 = Greater?(x=w654, y=w653) -> (0:→"Web Cam":bool)
    n161 = call "GrabWebCam_PCO_IOS.vi"("Session In"=w661, "Image In"=w662, "Trial Time"=w663, "AVI Refnum"=w658, "error in"=w660) -> ("Session Out"=w659:T7, "WebCam Img Out"=→"?":T3, "Buffer Number Out"=w657:u32, "error out"=w650:errorcluster)  [unwired: 7 in]
    n162 = local read "CBV Camera"() -> (w652:bool)
    n163 = local read "stop"() -> (w649:bool)
    n164 = call <vilib>:"Calculate Frames per Second.vi"("Update Interval (ms)"=u32 5000, "Buffer Number"=w657) -> ("Processed Frames/s"=→"Web Cam Fs":dbl)  [unwired: 7 in, 2 out]
    n165 = Compound Arithmetic op=OR(w650, w649, w652) -> (w651:bool)
  }
  n166 = while {
    tunnel: w418 -> [w720]
    tunnel: w416 -> [w676]
    tunnel: w415 -> [w719]
    tunnel: w236 -> [_]
    tunnel: w191 -> [w703]
    tunnel: w190 -> [w704]
    tunnel: w189 -> [w698]
    tunnel: w188 -> [w695]
    tunnel: w145 -> [w692]
    tunnel: w74 -> [w691]
    tunnel: w73 -> [w690]
    tunnel: [w680] -> w62
    tunnel: [w679] -> w63
    tunnel: [w672] -> w67
    tunnel: w64 -> [w672]
    tunnel: w41 -> [w669]
    tunnel: w40 -> [w670]
    tunnel: [w670] -> w39
    tunnel: [w669] -> w38
    stop <- w714 stop-if-true
    n167 = call-dynamic "isRecording.vi"("Camera in"=w691, "error in (no error)"=w690) -> ("Camera out"=w678:refnum<class "Camera.lvclass">, "recording"=→"PCO":bool, "error out"=w677:errorcluster)  [unwired: 11 in]
    n168 = Tick Count (ms)() -> (millisecond timer value=w723:u32)
    n169 = call-dynamic "getRecordedImageCount.vi"("Camera in"=w678, "error in (no error)"=w677) -> ("Camera out"=w684:refnum<class "Camera.lvclass">, "recorded_image_count"=w675:u32, "error out"=w683:errorcluster)  [unwired: 11 in]
    "Recorded Images" <- w675
    n170 = Multiply(x=w692, y=w675) -> (x*y=w715:dbl)
    n171 = Round Toward -Infinity(1:w715) -> (0:w709:dbl)
    n172 = Index Array(array=w703, index (row)=w709) -> (element=w702:bool[])  [unwired: 1 in]
    n173 = Index Array(array=w704, index (row)=w709) -> (element=w700:bool[])  [unwired: 1 in]
    n174 = Index Array(array=w698, index (row)=w709) -> (element=w697:bool[])  [unwired: 1 in]
    n175 = Index Array(array=w695, index (row)=w709) -> (element=w694:bool[])  [unwired: 1 in]
    n176 = Subtract(x=w723, y=w720) -> (x-y=w722:u32)
    n177 = local read "Image"() -> (w689:T3)
    n178 = Greater Or Equal?(x=w675, y=w676) -> (x >= y?=w681:bool)
    n179 = Multiply(x=w722, y=1.667e-05) -> (x*y=w721:dbl)
    n180 = call-dynamic "image.vi"("Camera in"=w684, "data_format"=T15."Mono16", "image_index"=u32 4294967295 ("dwImgIdx"), "error in (no error)"=w683) -> ("Camera out"=w680:refnum<class "Camera.lvclass">, "raw_image (U16)"=w688:u16[][], "error out"=w679:errorcluster)  [unwired: 4 in, 5 out]
    n181 = call "IMAQ ArrayToImage"("Image Pixels (U16)"=w688, "Image"=w689) -> ("error out"=w686:errorcluster, "Image Out"=w682:T3)  [unwired: 8 in]
    n182 = local write "stop"("stop") -> ()
    n183 = Bundle("Time (min)"=w719, w721) -> (→"Time Elapsed (Min)":cluster{"Time (min)":dbl, dbl})  [unwired: 1 in]
    n184 = Greater?(x=w702, y=FALSE ("Boolean")) -> (0:w701:bool[])
    n185 = Greater?(x=w700, y=FALSE ("Boolean")) -> (0:w699:bool[])
    n186 = Greater?(x=w697, y=FALSE ("Boolean")) -> (0:w696:bool[])
    n187 = Greater?(x=w694, y=FALSE ("Boolean")) -> (0:w693:bool[])
    n188 = Unbundle By Name(w679) -> ("status"=w673:bool)
    n189 = Unbundle By Name(w686) -> ("status"=w674:bool)
    n190 = local write "Image"(w682) -> ()
    n191 = Or Array Elements(Boolean array=w701) -> (logical OR=→"LPad":bool)
    n192 = Or Array Elements(Boolean array=w699) -> (logical OR=→"Auditory":bool)
    n193 = Or Array Elements(Boolean array=w696) -> (logical OR=→"RPad":bool)
    n194 = Or Array Elements(Boolean array=w693) -> (logical OR=→"LED":bool)
    n195 = Compound Arithmetic op=OR(w673, w674, w681, "stop") -> (w714:bool)
    "CBV Camera" <- w714
    "Finished" <- w714
  }
  n196 = while {
    tunnel: [w745] -> w134
    tunnel: [w746] -> w135
    tunnel: [w751] -> w130
    tunnel: w427 -> [w750]
    tunnel: w425 -> [w749]
    tunnel: w423 -> [w748]
    tunnel: w421 -> [w747]
    shift-right: [w736] -> _
    shift-left: _ -> [w734]
    shift-right: [w731] -> _
    shift-left: u32 0 ("New Lost") -> [w735]
    shift-right: [w732] -> w115
    shift-left: u32[] [] ("NewBuffNum") -> [w733]
    shift-right: [w738] -> w118
    shift-left: u32[] [] ("NewNumLost") -> [w737]
    tunnel: w268 -> [w743]
    tunnel: w236 -> [w739]
    tunnel: [w725] -> w50
    tunnel: w51 -> [w725]
    tunnel: w49 -> [w724]
    tunnel: [w724] -> w48
    i -> [w726]
    stop <- w742 stop-if-true
    n197 = call <vilib>:"IMAQdx Get Image.vi"("Buffer Number Mode (Next)"=IMAQdx_Buffer_Number_Mode."Buffer Number", "error in"=w749, "Buffer Number In"=w726, "Image In"=w748, "Session In"=w750) -> ("error out"=w757:errorcluster, "Buffer Number Out"=w736:u32, "Image Out"=w728:T3, "Session Out"=w745:T7)  [unwired: 3 in]
    "Last Whisk\nBuffer" <- w736
    "?" <- w728
    n198 = Greater?(x=w726, y=w739) -> (0:→"Whisk Cam":bool)
    n199 = call "IMAQ ImageToArray"("error in (no error)"=w757, "Image"=w728) -> ("error out"=w756:errorcluster, "Image Pixels (U8)"=w755:u8[][])  [unwired: 2 in, 3 out]
    n200 = call "TrackWhiskDroppedFrames_PCO_IOS.vi"("NumLost"=w737, "BuffNum"=w733, "Curr Buffer"=w736, "Prev Lost"=w735, "Prev Buffer"=w734) -> ("New Lost"=w731:u32, "NewNumLost"=w738:u32[], "NewBuffNum"=w732:u32[])  [unwired: 4 in]
    "Dropped" <- w731
    n201 = Add(x=w736, y=w735) -> (x+y=w744:u32)
    n202 = Greater Or Equal?(x=w744, y=w743) -> ()  [unwired: 1 out]
    n203 = Write to Binary File(file (use dialog)=w747, data=w755, error in=w756, 5:FALSE ("prepend array or string size? (T)"), 9:T16."little-endian" ("byte order (0:big-endian, network order)")) -> (refnum out=w751:refnum<file>, error out=w746:errorcluster)  [unwired: 1 in, 1 out]
    n204 = local read "stop"() -> (w730:bool)
    n205 = local read "CBV Camera"() -> (w729:bool)
    n206 = call <vilib>:"Calculate Frames per Second.vi"("Update Interval (ms)"=u32 2000, "Buffer Number"=w736) -> ("Processed Frames/s"=→"Whisk Cam Fs":dbl)  [unwired: 7 in, 2 out]
    n207 = Unbundle By Name(w746) -> ("status"=w727:bool)
    n208 = Compound Arithmetic op=OR(w727, w730, w729) -> (w742:bool)
  }
  n209 = while {
    tunnel: w172 -> [w759]
    tunnel: [w760] -> w157
    tunnel: w171 -> [w760]
    tunnel: [w759] -> w158
    stop <- w761 stop-if-true
    n210 = local read "Finished"() -> (w761:bool)
  }
  n211 = while {
    tunnel: [w776] -> w150
    tunnel: [w777] -> w149
    tunnel: [w786] -> w128
    tunnel: w283 -> [w785]
    tunnel: w282 -> [w784]
    tunnel: w277 -> [w783]
    tunnel: w281 -> [w782]
    shift-right: [w775] -> _
    shift-left: _ -> [w781]
    shift-right: [w780] -> _
    shift-left: u32 0 ("New Lost") -> [w774]
    shift-right: [w779] -> w109
    shift-left: u32[] [] ("NewBuffNum") -> [w770]
    shift-right: [w778] -> w112
    shift-left: u32[] [] ("NewNumLost") -> [w771]
    tunnel: w267 -> [w769]
    tunnel: w236 -> [w767]
    i -> [w762]
    stop <- w772 stop-if-true
    n212 = call <vilib>:"IMAQdx Get Image.vi"("Buffer Number Mode (Next)"=IMAQdx_Buffer_Number_Mode."Buffer Number", "error in"=w784, "Buffer Number In"=w762, "Image In"=w783, "Session In"=w785) -> ("error out"=w793:errorcluster, "Buffer Number Out"=w775:u32, "Image Out"=w764:T3, "Session Out"=w776:T7)  [unwired: 3 in]
    "Last Whisk\nBuffer 2" <- w775
    "?" <- w764
    n213 = Greater?(x=w762, y=w767) -> (0:→"Pupil Cam":bool)
    n214 = call "TrackPupilDroppedFrames_PCO_IOS.vi"("NumLost"=w771, "BuffNum"=w770, "Curr Buffer"=w775, "Prev Lost"=w774, "Prev Buffer"=w781) -> ("New Lost"=w780:u32, "NewNumLost"=w778:u32[], "NewBuffNum"=w779:u32[])  [unwired: 4 in]
    "Dropped 2" <- w780
    n215 = call "IMAQ ImageToArray"("error in (no error)"=w793, "Image"=w764) -> ("error out"=w792:errorcluster, "Image Pixels (U8)"=w791:u8[][])  [unwired: 2 in, 3 out]
    n216 = Add(x=w775, y=w774) -> (x+y=w773:u32)
    n217 = Greater Or Equal?(x=w773, y=w769) -> ()  [unwired: 1 out]
    n218 = Write to Binary File(file (use dialog)=w782, data=w791, error in=w792, 5:FALSE ("prepend array or string size? (T)"), 9:T16."little-endian" ("byte order (0:big-endian, network order)")) -> (refnum out=w786:refnum<file>, error out=w777:errorcluster)  [unwired: 1 in, 1 out]
    n219 = local read "stop"() -> (w766:bool)
    n220 = local read "CBV Camera"() -> (w765:bool)
    n221 = call <vilib>:"Calculate Frames per Second.vi"("Update Interval (ms)"=u32 2000, "Buffer Number"=w775) -> ("Processed Frames/s"=→"Pupil Cam Fs":dbl)  [unwired: 7 in, 2 out]
    n222 = Unbundle By Name(w777) -> ("status"=w763:bool)
    n223 = Compound Arithmetic op=OR(w763, w766, w765) -> (w772:bool)
  }
  n224 = flat-sequence {
    tunnel: w158 -> [w836]
    tunnel: w157 -> [w835]
    tunnel: [w834] -> w156
    tunnel: [w833] -> w155
    tunnel: [w832] -> w154
    tunnel: [w831] -> w153
    tunnel: [w830] -> w151
    tunnel: w150 -> [w830]
    tunnel: w149 -> [w818]
    tunnel: [w818] -> w148
    tunnel: w144 -> [w829]
    tunnel: w143 -> [w817]
    tunnel: [w828] -> w142
    tunnel: [w827] -> w141
    tunnel: w140 -> [w825]
    tunnel: w139 -> [w826]
    tunnel: w138 -> [w824]
    tunnel: [w823] -> w137
    tunnel: w135 -> [w821]
    tunnel: w134 -> [w822]
    tunnel: [w821] -> w132
    tunnel: [w820] -> w131
    tunnel: w130 -> [w820]
    tunnel: w128 -> [w819]
    tunnel: [w819] -> w127
    tunnel: [w818] -> w124
    tunnel: [w817] -> w123
    tunnel: w120 -> [w816]
    tunnel: [w816] -> w121
    tunnel: w118 -> [w815]
    tunnel: [w815] -> w117
    tunnel: w115 -> [w814]
    tunnel: [w814] -> w114
    tunnel: w112 -> [w813]
    tunnel: [w813] -> w111
    tunnel: w109 -> [w812]
    tunnel: [w812] -> w108
    tunnel: w105 -> [w811]
    tunnel: [w811] -> w104
    tunnel: w67 -> [w810]
    tunnel: [w810] -> w66
    tunnel: w63 -> [w809]
    tunnel: w62 -> [w808]
    tunnel: [w804] -> w55
    tunnel: [w803] -> w54
    tunnel: w52 -> [w802]
    tunnel: w53 -> [w801]
    tunnel: w50 -> [w798]
    tunnel: w48 -> [w800]
    tunnel: [w799] -> w47
    tunnel: [w797] -> w46
    tunnel: w39 -> [w796]
    tunnel: w38 -> [w795]
    tunnel: w156 -> [w867]
    tunnel: w155 -> [w866]
    tunnel: w154 -> [w865]
    tunnel: w153 -> [w864]
    tunnel: w151 -> [w863]
    tunnel: w148 -> [w862]
    tunnel: w142 -> [w861]
    tunnel: w141 -> [w860]
    tunnel: w137 -> [w859]
    tunnel: [w859] -> w136
    tunnel: [w858] -> w133
    tunnel: w132 -> [w858]
    tunnel: w131 -> [w857]
    tunnel: [w857] -> w129
    tunnel: w127 -> [w856]
    tunnel: [w856] -> w126
    tunnel: [w855] -> w125
    tunnel: w124 -> [w855]
    tunnel: w123 -> [w854]
    tunnel: [w854] -> w122
    tunnel: w121 -> [w853]
    tunnel: [w853] -> w119
    tunnel: w117 -> [w852]
    tunnel: [w852] -> w116
    tunnel: [w851] -> w113
    tunnel: w114 -> [w851]
    tunnel: w111 -> [w850]
    tunnel: [w850] -> w110
    tunnel: w108 -> [w849]
    tunnel: [w849] -> w107
    tunnel: [w848] -> w106
    tunnel: w104 -> [w848]
    tunnel: "Target Path" -> [w846]
    tunnel: w66 -> [w842]
    tunnel: w55 -> [w840]
    tunnel: w54 -> [w839]
    tunnel: w47 -> [w838]
    tunnel: w46 -> [w837]
    frame #0 {
      n225 = call-poly <vilib>:"DAQmx Write.vi"("task/channels in"=w801, "data"=FALSE, "error in"=w802) -> ("task out"=w806:refnum<k21>, "error out"=w807:errorcluster)  [unwired: 10 in, 1 out]
      n226 = call-dynamic "close.vi"("error in (no error)"=w809, "Camera in"=w808) -> ()  [unwired: 9 in, 1 out]
      n227 = call <vilib>:"DAQmx Stop Task.vi"("task/channels in"=w798, "error in"=w800) -> ("task out"=w797:refnum<k21>, "error out"=w799:errorcluster)  [unwired: 12 in]
      n228 = call <vilib>:"DAQmx Stop Task.vi"("task/channels in"=w836, "error in"=w835) -> ("task out"=w834:refnum<k21>, "error out"=w833:errorcluster)  [unwired: 12 in]
      n229 = call <vilib>:"DAQmx Stop Task.vi"("task/channels in"=w796, "error in"=w795) -> ("task out"=w832:refnum<k21>, "error out"=w831:errorcluster)  [unwired: 12 in]
      n230 = call <vilib>:"IMAQdx Close Camera.vi"("error in"=w821, "Session In"=w822) -> ()  [unwired: 9 in, 1 out]
      n231 = call "IMAQ AVI2 Close"("error in (no error)"=w825, "AVI Refnum"=w824) -> ("error out"=w823:errorcluster)  [unwired: 9 in]
      n232 = call <vilib>:"IMAQdx Close Camera.vi"("error in"=w825, "Session In"=w826) -> ()  [unwired: 9 in, 1 out]
      n233 = call <vilib>:"DAQmx Stop Task.vi"("task/channels in"=w829, "error in"=w817) -> ("task out"=w828:refnum<k21>, "error out"=w827:errorcluster)  [unwired: 12 in]
      n234 = call <vilib>:"DAQmx Stop Task.vi"("task/channels in"=w806, "error in"=w807) -> ("task out"=w803:refnum<k21>, "error out"=w804:errorcluster)  [unwired: 12 in]
    }
    frame #1 {
      n235 = Path To String(path=w842) -> (string=w845:string)
      n236 = call <vilib>:"DAQmx Clear Task.vi"("task in"=w839, "error in"=w840) -> ()  [unwired: 13 in, 1 out]
      n237 = call <vilib>:"DAQmx Clear Task.vi"("task in"=w867, "error in"=w866) -> ()  [unwired: 13 in, 1 out]
      n238 = call <vilib>:"DAQmx Clear Task.vi"("task in"=w865, "error in"=w864) -> ()  [unwired: 13 in, 1 out]
      n239 = call <vilib>:"IMAQdx Close Camera.vi"("error in"=w862, "Session In"=w863) -> ()  [unwired: 9 in, 1 out]
      n240 = call <vilib>:"DAQmx Clear Task.vi"("task in"=w837, "error in"=w838) -> ()  [unwired: 13 in, 1 out]
      n241 = call <vilib>:"DAQmx Clear Task.vi"("task in"=w861, "error in"=w860) -> ()  [unwired: 13 in, 1 out]
      n242 = Concatenate Strings(w845, "_Cam01.pcoraw" ("string")) -> (w843:string)
      n243 = String To Path(string=w843) -> (path=w841:path)
      n244 = Move(source path=w841, 10:w846) -> (error out=w847:errorcluster)  [unwired: 3 in, 2 out]
      n245 = call <vilib>:"Simple Error Handler.vi"("error in (no error)"=w847) -> ()  [unwired: 1 in, 8 out]
    }
  }
  n246 = Delete From Array(array=w113, length=1, index=0) -> (array with subset deleted=w322:u32[])  [unwired: 1 out]
  n247 = Delete From Array(array=w116, length=1, index=0) -> (array with subset deleted=w323:u32[])  [unwired: 1 out]
  n248 = Delete From Array(array=w110, length=1, index=0) -> (array with subset deleted=w254:u32[])  [unwired: 1 out]
  n249 = Delete From Array(array=w107, length=1, index=0) -> (array with subset deleted=w253:u32[])  [unwired: 1 out]
  n250 = Close File(refnum=w129, error in=w133) -> (path=w398:path, error out=w397:errorcluster)
  n251 = Close File(refnum=w126, error in=w125) -> (path=w250:path, error out=w249:errorcluster)
  n252 = Build Array(w322, w323) -> (w325:u32[][])
  n253 = Build Array(w253, w254) -> (w256:u32[][])
  n254 = Array To Spreadsheet String(delimiter (Tab)=",", array=w323, 3:"%d" ("format string")) -> (spreadsheet string=w331:string)
  n255 = Transpose 2D Array(2D array=w325) -> (transposed array=w324:u32[][])
  n256 = Array To Spreadsheet String(delimiter (Tab)=",", array=w322, 3:"%d" ("format string")) -> (spreadsheet string=w332:string)
  n257 = Move(source path=w250, error in=w249, 10:"Target Path") -> (error out=w251:errorcluster)  [unwired: 2 in, 2 out]
  n258 = Move(source path=w398, error in=w397, 10:"Target Path") -> (error out=w395:errorcluster)  [unwired: 2 in, 2 out]
  n259 = Array To Spreadsheet String(delimiter (Tab)=",", array=w254, 3:"%d" ("format string")) -> (spreadsheet string=w257:string)
  n260 = Transpose 2D Array(2D array=w256) -> (transposed array=w255:u32[][])
  n261 = Move(source path=w106, error in=w136, 10:"Target Path") -> (error out=w394:errorcluster)  [unwired: 2 in, 2 out]
  n262 = Array To Spreadsheet String(delimiter (Tab)=",", array=w253, 3:"%d" ("format string")) -> (spreadsheet string=w258:string)
  n263 = call <vilib>:"Trim Whitespace.vi"("string"=w332) -> ("trimmed string"=w244:string)  [unwired: 1 in]
  n264 = call <vilib>:"Trim Whitespace.vi"("string"=w331) -> ("trimmed string"=w243:string)  [unwired: 1 in]
  n265 = Number To Decimal String(number=w324) -> ()  [unwired: 1 in, 1 out]
  n266 = call <vilib>:"Trim Whitespace.vi"("string"=w258) -> ("trimmed string"=w245:string)  [unwired: 1 in]
  n267 = call <vilib>:"Trim Whitespace.vi"("string"=w257) -> ("trimmed string"=w246:string)  [unwired: 1 in]
  n268 = Number To Decimal String(number=w255) -> ()  [unwired: 1 in, 1 out]
  n269 = call <vilib>:"Simple Error Handler.vi"("error in (no error)"=w251) -> ()  [unwired: 1 in, 8 out]
  n270 = call <vilib>:"Simple Error Handler.vi"("error in (no error)"=w395) -> ()  [unwired: 1 in, 8 out]
  n271 = call <vilib>:"Simple Error Handler.vi"("error in (no error)"=w394) -> ()  [unwired: 1 in, 8 out]
  n272 = Build Array(w245, w246, w244, w243) -> (w242:string[])
  n273 = TDMS Set Properties(5:w242, 7:string[] ["PupilCam_DroppedFrameIndex", "PupilCam_NumberDropped", "WhiskCam_DroppedFrameIndex", "WhiskCam_NumberDropped"] ("channel name(s) in (Untitled)"), 8:w122, 11:w119) -> (0:w338:errorcluster, 3:w337:refnum<k34>)  [unwired: 2 in, 2 out]
  n274 = TDMS Close(8:w338, 11:w337) -> (0:w399:errorcluster, 3:w391:path)
  n275 = Path To String(path=w391) -> (string=w393:string)
  n276 = TDMS Defragment(4:w399, 7:w391) -> (0:w388:errorcluster)
  n277 = Concatenate Strings(w393, "_index" ("string")) -> (w390:string)
  n278 = String To Path(string=w390) -> (path=w389:path)
  n279 = Move(source path=w391, error in=w388, 10:"Target Path") -> (error out=w396:errorcluster)  [unwired: 2 in, 2 out]
  n280 = Move(source path=w389, error in=w388, 10:"Target Path") -> (error out=w252:errorcluster)  [unwired: 2 in, 2 out]
  n281 = call <vilib>:"Simple Error Handler.vi"("error in (no error)"=w396) -> ()  [unwired: 1 in, 8 out]
  n282 = call <vilib>:"Simple Error Handler.vi"("error in (no error)"=w252) -> ()  [unwired: 1 in, 8 out]
